vi "Button_Create.vi"(0 "reference in":refnum<class "Button.lvclass">, 11 "Error In":errorcluster) -> (4 "reference out":refnum<class "Button.lvclass">, 15 "Error Out":errorcluster)   [LabVIEW 2024, in "Button.lvclass"]
uses:
  Button.lvclass
  Button.lvclass/Button.ctl
panel:
  # "Connector Pane"
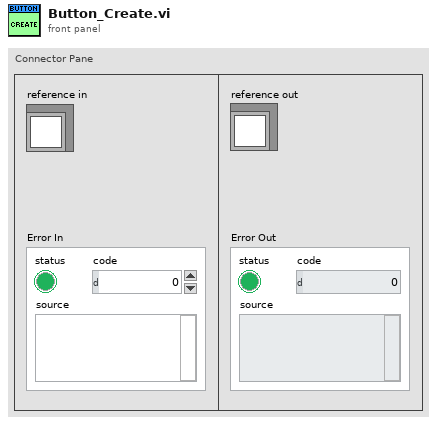
[diagram p1: front panel]
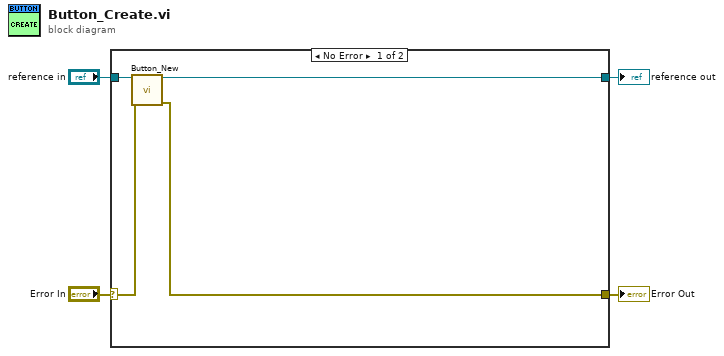
[diagram p0: block diagram]
diagram:
  n1 = case shown="No Error" "Error In" {
    selector: "Error In" -> [w7 w10]
    tunnel: [w5 w10] -> w3
    tunnel: "reference in" -> [w8 w9]
    tunnel: [w6 w9] -> w1
    frame No Error {
      n2 = call "Button_New.vi"("reference in"=w8, "Error In"=w7) -> ("reference out"=w6:refnum<class "Button.lvclass">, "Error Out"=w5:errorcluster)  [unwired: 10 in, 2 out]
    }
    frame Error {
      # "VI-TechBaseTemplate_Simple_4x4x4"
    }
  }
  "Error Out" <- w3
  "reference out" <- w1
